vi "Test Reducing Memory Footprint.vi"() -> ()   [LabVIEW 2011]
panel:
  out "x-y":u32
  out "Image":T1(plugin-control)
  in  "stop":bool
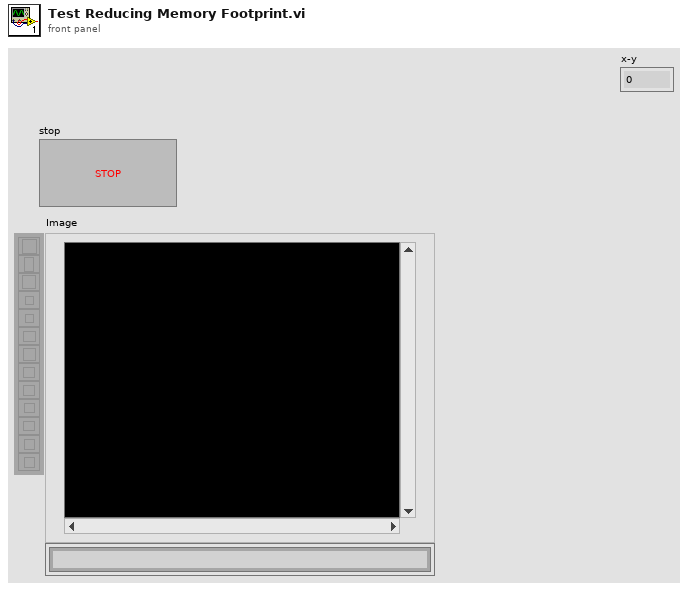
[diagram p1: front panel]
types:
  T1 = typedef "IMAQ Image.ctl" = refnum<image>
  T2 = typedef "Image Type" = u32
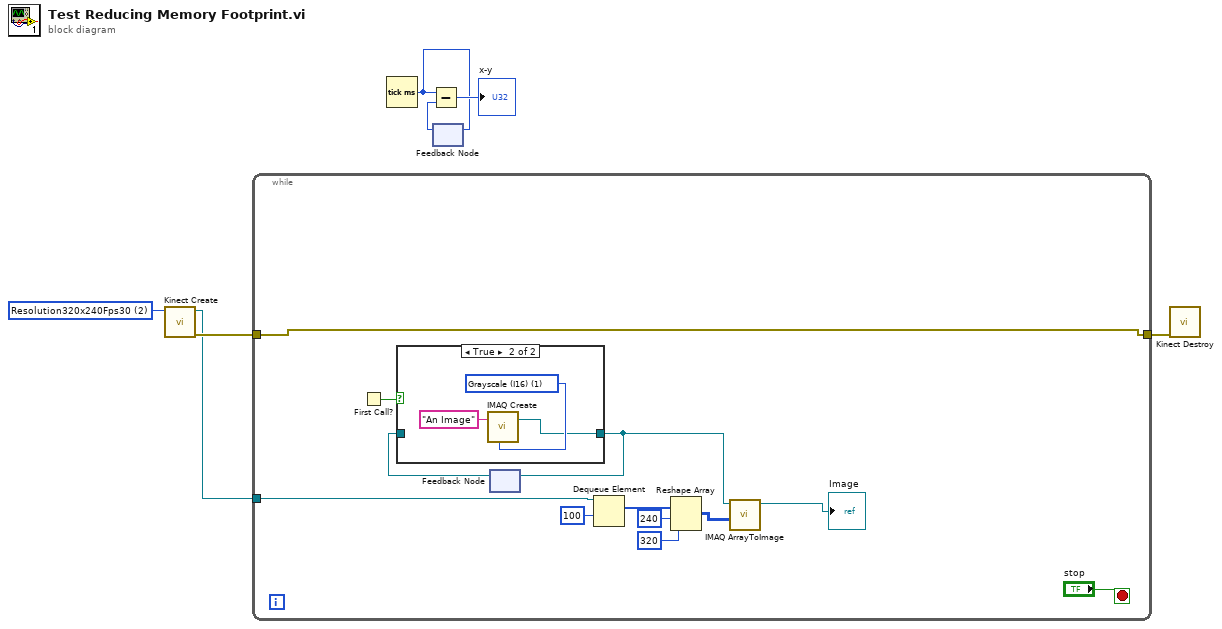
[diagram p0: block diagram]
diagram:
  w6 = 2 items=["Undefined", "Resolution640x480Fps30", "Resolution320x240Fps30", "Resolution80x60Fps30"] ("Depth Format")
  n1 = call "Kinect Create.vi"("Depth Format"=w6) -> ("error out"=w7:errorcluster, "queue out"=w1:refnum<queue>)  [unwired: 9 in]
  n2 = while {
    tunnel: w7 -> [w8]
    tunnel: w1 -> [w9]
    tunnel: [w8] -> w2
    stop <- "stop" stop-if-true
    n3 = First Call?() -> (First Call?: T/F=w13:bool)
    n4 = feedback #1() -> (w11:T1)  [unwired: 1 in]
    n5 = case shown="True" w13 {
      tunnel: [w20 w21] -> w12
      tunnel: w11 -> [w20 _]
      frame False {
      }
      frame True {
        w22 = T2 1 items=["Grayscale (U8)", "Grayscale (I16)", "Grayscale (SGL)", "Complex (CSG)", "RGB (U32)", "HSL (U32)", "RGB (U64)", "Grayscale (U16)"] ("Image Type")
        n6 = call "IMAQ Create"("Image Name"="An Image", "Image Type"=w22) -> ("New Image"=w21:T1)  [unwired: 3 in, 1 out]
      }
    }
    n7 = feedback-in #1(w12) -> ()
    n8 = Dequeue Element(queue=w9, timeout in ms (-1)=100) -> (element=w18:i16[])  [unwired: 1 in, 3 out]
    n9 = Reshape Array(w18, 240 ("dimension size"), 320 ("dimension size")) -> (w15:i16[][])
    n10 = call "IMAQ ArrayToImage"("Image Pixels (I16)"=w15, "Image"=w12) -> ("Image Out"=→"Image":T1)  [unwired: 8 in, 1 out]
  }
  n11 = Tick Count (ms)() -> (millisecond timer value=w3:u32)
  n12 = feedback #2() -> (w4:u32)  [unwired: 1 in]
  n13 = Subtract(x=w3, y=w4) -> (x-y=→"x-y":u32)
  n14 = feedback-in #2(w3) -> ()
  n15 = call "Kinect Destroy.vi"("error in"=w2) -> ()  [unwired: 10 in, 1 out]
